vi "6.vi"() -> ()   [LabVIEW 2020]
uses:
  #typedef_Student.ctl
  #typedef_6Action.ctl
  #typedef_DatabaseAction.ctl
panel:
  in  "Student":T1
  out "Database":T1[](array[typedef])
  in  "Exit":bool
  in  "Clear Database":bool
  in  "Get Database":bool
  in  "Add User":bool
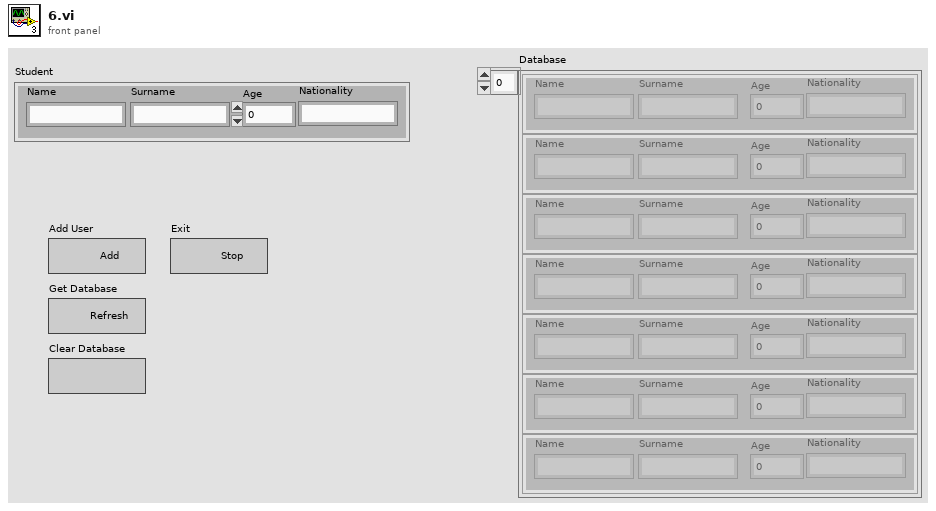
[diagram p1: front panel]
types:
  T1 = typedef "#typedef_Student.ctl" = cluster{"Name":string, "Surname":string, "Age":dbl, "Nationality":string}
  T2 = typedef "#typedef_6Action.ctl" = enum16{"Initialize", "Idle", "Add User", "Get Database", "Clear Database", "Exit"}
  T3 = typedef "#typedef_DatabaseAction.ctl" = enum16{"Add user", "Get database", "Clear database"}
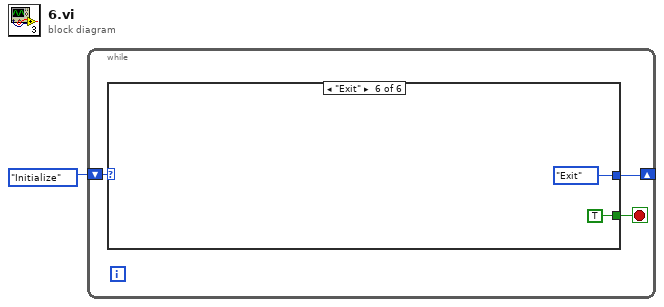
[diagram p0: block diagram]
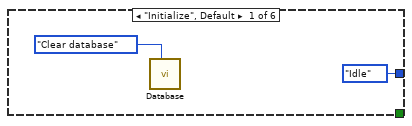
[diagram p2: hidden frame]
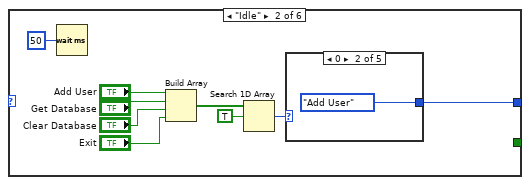
[diagram p3: hidden frame]
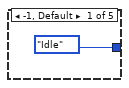
[diagram p4: hidden frame]
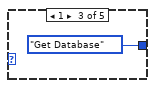
[diagram p5: hidden frame]
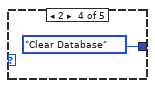
[diagram p6: hidden frame]
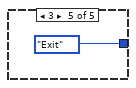
[diagram p7: hidden frame]
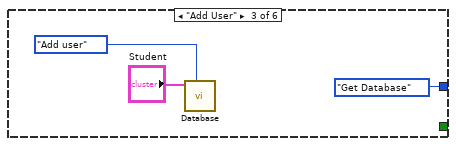
[diagram p8: hidden frame]
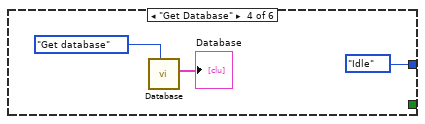
[diagram p9: hidden frame]
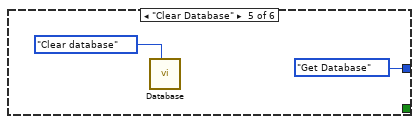
[diagram p10: hidden frame]
diagram:
  n1 = while {
    shift-right: [w3] -> _
    shift-left: #typedef_6Action."Initialize" ("6_Action") -> [w4]
    stop <- w2 stop-if-true
    n2 = case shown="\"Exit\"" w4 {
      tunnel: [#typedef_6Action."Idle" ("6_Action") w10 #typedef_6Action."Get Database" ("6_Action") #typedef_6Action."Idle" ("6_Action") #typedef_6Action."Get Database" ("6_Action") #typedef_6Action."Exit" ("6_Action")] -> w3
      tunnel: [_ _ _ _ _ TRUE] -> w2
      frame "Initialize", Default {
        n3 = call "Database.vi"("Database Action"=#typedef_DatabaseAction."Clear database") -> ()  [unwired: 10 in, 1 out]
      }
      frame "Idle" {
        n4 = Wait (ms)(milliseconds to wait=u32 50) -> ()  [unwired: 1 out]
        n5 = Build Array("Add User", "Get Database", "Clear Database", "Exit") -> (w13:bool[])
        n6 = Search 1D Array(1D array=w13, element=TRUE) -> (index of element=w11:i32)  [unwired: 1 in]
        n7 = case shown="0" w11 {
          tunnel: [#typedef_6Action."Idle" ("6_Action") #typedef_6Action."Add User" ("6_Action") #typedef_6Action."Get Database" ("6_Action") #typedef_6Action."Clear Database" ("6_Action") #typedef_6Action."Exit" ("6_Action")] -> w10
          frame -1, Default {
          }
          frame 0 {
          }
          frame 1 {
          }
          frame 2 {
          }
          frame 3 {
          }
        }
      }
      frame "Add User" {
        n8 = call "Database.vi"("Database Action"=#typedef_DatabaseAction."Add user", "User"="Student") -> ()  [unwired: 9 in, 1 out]
      }
      frame "Get Database" {
        n9 = call "Database.vi"("Database Action"=#typedef_DatabaseAction."Get database") -> ("Database"=→"Database":T1[])  [unwired: 10 in]
      }
      frame "Clear Database" {
        n10 = call "Database.vi"("Database Action"=#typedef_DatabaseAction."Clear database") -> ()  [unwired: 10 in, 1 out]
      }
      frame "Exit" {
      }
    }
  }
